vi "CH_LM Config Gain Compensation.vi"(0 "Meter Index":i32, 1 "Compensation Factor (1.0)":dbl=1.0 format="%#.3g", 5 "error in (no error)":errorcluster, 7 "Timeout / ms (3000)":i32=3000, 8 "Action (query)":bool, 9 "Lock Timeout / ms (1000)":i32=1000) -> (11 "Lock timed out":bool, 14 "Meter Index":i32, 15 "Compensation Factor":dbl format="%#.3g", 19 "error out":errorcluster)   [LabVIEW 2012, in "CH_LM.lvlib"]
doc: "This VI will set/query the gain compensation factor. The gain compensation factor has no units."
uses:
  CH_LM.lvlib
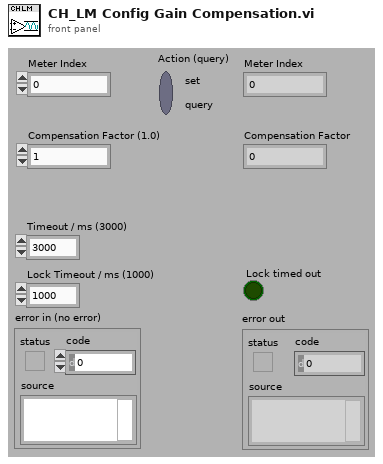
[diagram p1: front panel]
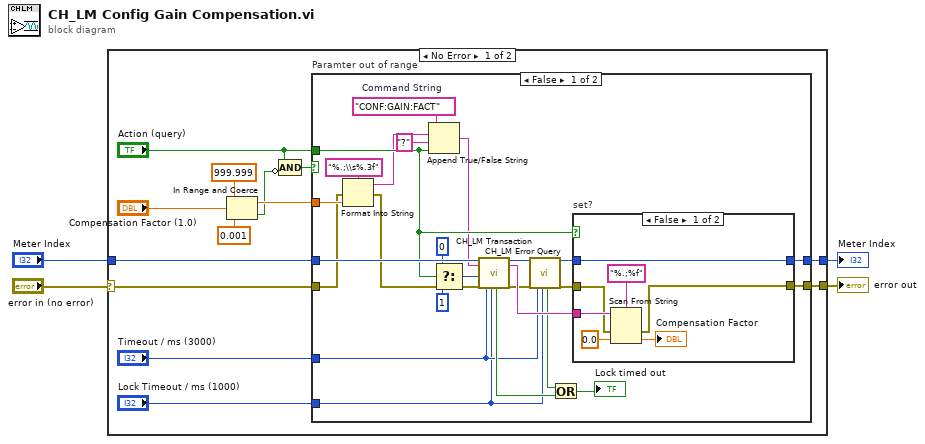
[diagram p0: block diagram]
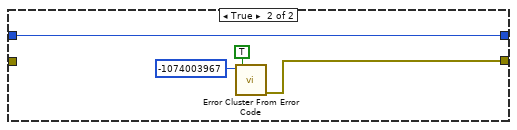
[diagram p3: hidden frame]
diagram:
  n1 = case shown="No Error" "error in (no error)" {
    selector: "error in (no error)" -> [w17 w57]
    tunnel: [w15 w57] -> w4
    tunnel: "Meter Index" -> [w16 w56]
    tunnel: [w14 w56] -> w1
    frame No Error {
      n2 = In Range and Coerce(upper limit=999.999, x="Compensation Factor (1.0)", lower limit=0.001) -> (coerced(x)=w10:dbl, In Range?=w7:bool)
      n3 = Compound Arithmetic op=AND("Action (query)", invert w7) -> (w5:bool)
      n4 = case "Paramter out of range" shown="False" w5 {
        tunnel: w17 -> [w21 _]
        tunnel: w16 -> [w42 w55]
        tunnel: [w39 w53] -> w15
        tunnel: [w33 w55] -> w14
        tunnel: "Timeout / ms (3000)" -> [w25 _]
        tunnel: "Lock Timeout / ms (1000)" -> [w24 _]
        tunnel: w10 -> [w22 _]
        tunnel: "Action (query)" -> [w23 _]
        frame False {
          w41 = "CONF:GAIN:FACT"  # Command String
          n5 = Format Into String(format string="%.;\\s%.3f", error in=w21, w22) -> (resulting string=w18:string, error out=w20:errorcluster)  [unwired: 1 in]
          n6 = Append True/False String(1:w23, 2:"?" ("true string"), 3:w18, 4:w41) -> (0:w19:string)
          n7 = Select(t=0, s=w23, f=1 ("NofStrings (-1:all)")) -> (s? t:f=w35:i32)
          n8 = call "CH_LM Transaction.vi"("Meter Index"=w42, "Command String"=w19, "NofStrings (-1:all)"=w35, "error in (no error)"=w20, "Timeout / ms (3000)"=w25, "Lock Timeout / ms (1000)"=w24) -> ("Lock timed out"=w27:bool, "Meter Index"=w32:i32, "Response"=w40:string, "error out"=w30:errorcluster)  [unwired: 10 out]
          n9 = call "CH_LM Error Query.vi"("Meter Index"=w32, "error in (no error)"=w30, "Timeout / ms (3000)"=w25, "Lock Timeout / ms (1000)"=w24) -> ("Lock timed out"=w28:bool, "Meter Index"=w31:i32, "error out"=w29:errorcluster)  [unwired: 13 out]
          n10 = Or(x=w28, y=w27) -> (x .or. y?=→"Lock timed out":bool)
          n11 = case "set?" shown="False" w23 {
            tunnel: w40 -> [w49 _]
            tunnel: w29 -> [w48 w51]
            tunnel: [w47 w51] -> w39
            tunnel: w31 -> [w43 w50]
            tunnel: [w43 w50] -> w33
            frame False {
              n12 = Scan From String(format string="%.;%f", input string=w49, error in=w48, default 1=0.0 ("default value 1")) -> (error out=w47:errorcluster, output 1=→"Compensation Factor":dbl)  [unwired: 1 in, 2 out]
            }
            frame True {
            }
          }
        }
        frame True {
          n13 = call <vilib>:"Error Cluster From Error Code.vi"("show call chain? (False)"=TRUE, "error code (0)"=-1074003967) -> ("error out"=w53:errorcluster)  [unwired: 1 in, 6 out]
        }
      }
    }
    frame Error {
    }
  }
  "error out" <- w4
  "Meter Index" <- w1
